vi "Close Hardware.vi"(8 "error in (no error)":errorcluster, 11 "Instrument.Template in":refnum<class "Instrument.Element2.lvclass">) -> (0 "error out":errorcluster, 3 "Instrument.Template out":refnum<class "Instrument.Element2.lvclass">)   [LabVIEW 2019, in "Instrument.Element2.lvclass"]
uses:
  Instrument.Element2.lvclass
  Instrument.Element2.lvclass/Instrument.Element2.ctl
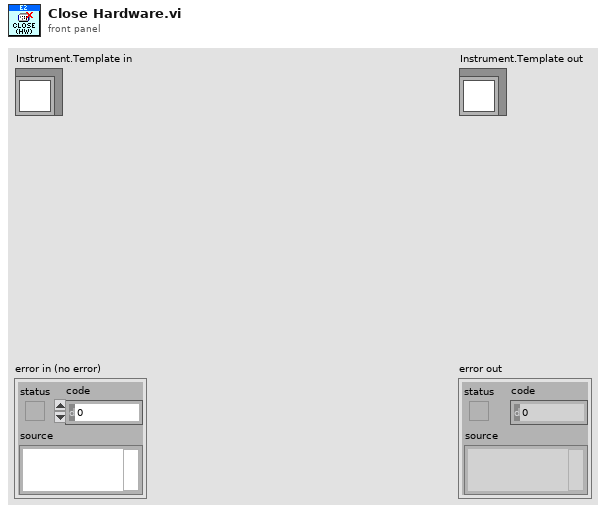
[diagram p1: front panel]
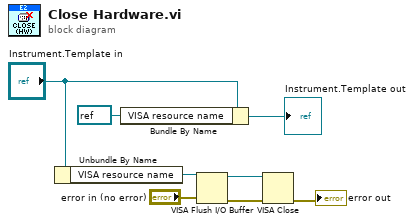
[diagram p0: block diagram]
diagram:
  n1 = Unbundle By Name("Instrument.Template in") -> ("VISA resource name"=w1:refnum<visa-resource-name>)
  n2 = Bundle By Name(cluster="Instrument.Template in", "VISA resource name"=refnum<visa-resource-name> refnum) -> (→"Instrument.Template out":refnum<class "Instrument.Element2.lvclass">)
  n3 = VISA Flush I/O Buffer(VISA resource name=w1, error in (no error)="error in (no error)") -> (VISA resource name out=w8:refnum<visa-resource-name>, error out=w7:errorcluster)  [unwired: 1 in]
  n4 = VISA Close(VISA resource name=w8, error in (no error)=w7) -> (error out=→"error out":errorcluster)
